vi "LabVLC - SpeedControl.vi"(2 "error in (no error)":errorcluster, 3 "video_speed":sgl(slide) min=0 max=2 step=0.1 scale=0.0..2.0, 4 "LabVLC":T1={"media_ptr"=0, "vlc_inst_ptr"=0, "path in"=path "C:/Program Files (x86)/VideoLAN/VLC/libvlc.dll"}) -> (0 "error out":errorcluster, 1 "LabVLC":T1)   [LabVIEW 2014]
doc: "Controls LabVLC playback speed. 1 is default. Numbers are decimal representations of percentages. You may double the speed by approaching 2, or halve the speed at 0.5. Single percision, floating-point representation for the input only. Requires a LabVLC cluster."
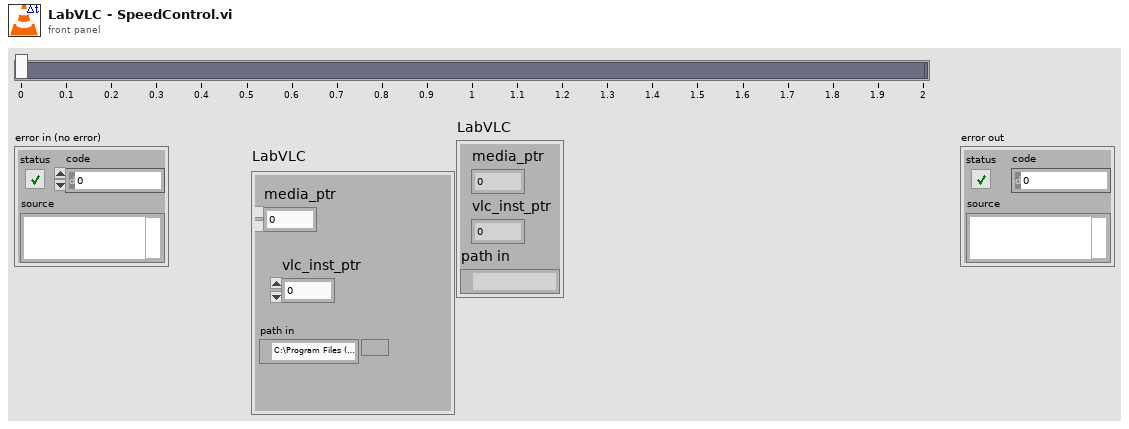
[diagram p1: front panel]
types:
  T1 = cluster{"media_ptr":i32, "vlc_inst_ptr":i32, "path in":path}
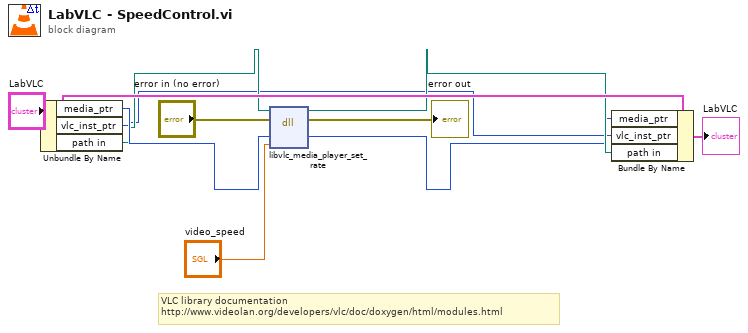
[diagram p0: block diagram]
diagram:
  # "VLC library documentation\nhttp://www.videolan.org/developers/vlc/doc/doxygen/html/modules.html"
  n1 = Unbundle By Name("LabVLC") -> ("media_ptr"=w6:i32, "vlc_inst_ptr"=w1:i32, "path in"=w5:path)
  n2 = dll-call lib="C:/Program Files (x86)/VideoLAN/VLC/libvlc.dll" fn="libvlc_media_player_set_rate"(path in=w5, error in="error in (no error)", "p_mi"=w6, "rate"="video_speed") -> (path out=w4:path, error out=→"error out":errorcluster, "p_mi"=w3:i32)  [unwired: 3 in]
  n3 = Bundle By Name(cluster="LabVLC", "media_ptr"=w3, "vlc_inst_ptr"=w1, "path in"=w4) -> (→"LabVLC":T1)
